vi "Test Set Subpanels-- SMO Array -- Started -- Duplicates.vi"(8 "error in":errorcluster) -> (0 "error out":errorcluster)   [LabVIEW 2020]
uses:
  Maui 2.0/Maui 2.0.lvclass
  C:/Program Files (x86)/National Instruments/LabVIEW 2020/vi.lib/JKI/JKI SMO/SMO/SMO.lvclass
  <vilib>/addons/_JKI Toolkits/Caraya/classes/Assert/Assert Equal Value_Variant.vi
  <vilib>/addons/_JKI Toolkits/Caraya/classes/Test/Test.lvclass
  <vilib>/JKI/JKI SMO/SMO/SMO.lvclass
  C:/Users/Albro/Documents/GitHub/MAUI-Engine/lvsrc/Maui 2.0/Maui 2.0/Maui 2.0.lvclass
  <vilib>/addons/_JKI Toolkits/Caraya/classes/Assert/Assert.lvclass
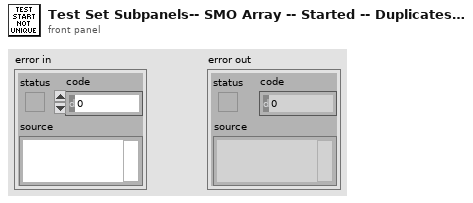
[diagram p1: front panel]
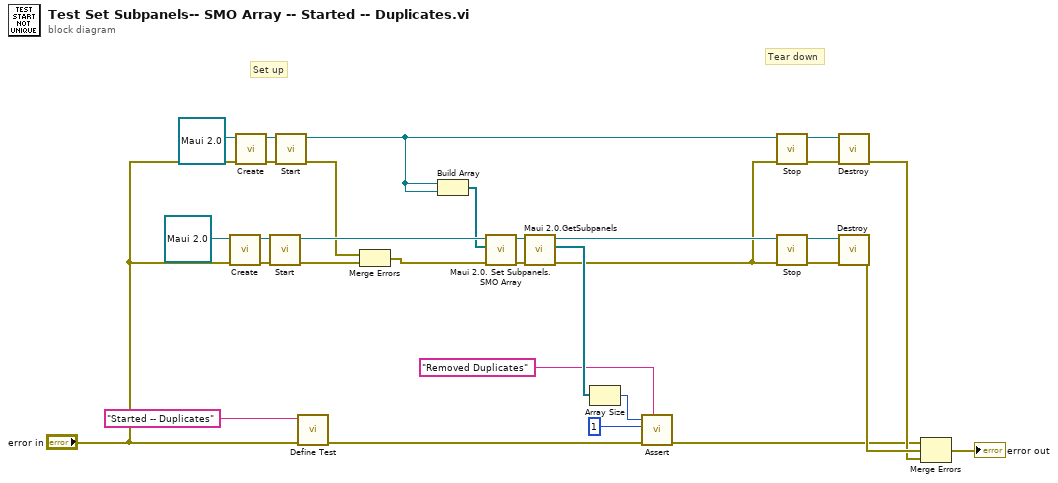
[diagram p0: block diagram]
diagram:
  # "Tear down"
  # "Set up"
  n1 = call <vilib>:"Create.vi"("error in (no error)"="error in", "SMO"=refnum<class "Maui 2.0.lvclass"> refnum ("Maui 2.0.lvclass")) -> ("error out"=w29:errorcluster, "SMO out"=w28:refnum<class "Maui 2.0.lvclass">)  [unwired: 7 in, 1 out]
  n2 = call <vilib>:"Create.vi"("error in (no error)"="error in", "SMO"=refnum<class "Maui 2.0.lvclass"> refnum ("Maui 2.0.lvclass")) -> ("error out"=w19:errorcluster, "SMO out"=w20:refnum<class "Maui 2.0.lvclass">)  [unwired: 7 in, 1 out]
  n3 = call <vilib>:"Start.vi"("error in (no error)"=w29, "SMO"=w28) -> ("error out"=w2:errorcluster, "SMO out"=w26:refnum<class "Maui 2.0.lvclass">)  [unwired: 8 in]
  n4 = call <vilib>:"Start.vi"("error in (no error)"=w19, "SMO"=w20) -> ("error out"=w3:errorcluster, "SMO out"=w12:refnum<class "Maui 2.0.lvclass">)  [unwired: 8 in]
  n5 = call <vilib>:"Define Test.vi"("error in (no error)"="error in", "Label (VI Title)"="Started -- Duplicates") -> ("error out"=w18:errorcluster)  [unwired: 9 in]
  n6 = Merge Errors(w3, w2) -> (w1:errorcluster)
  n7 = Build Array(w12, w12) -> (w13:refnum<class "Maui 2.0.lvclass">[])
  n8 = call-dynamic "Maui 2.0. Set Subpanels.SMO Array.vi"("error in (no error)"=w1, "Subpanels"=w13, "Maui 2.0 in"=w26) -> ("error out"=w15:errorcluster, "Maui 2.0 out"=w17:refnum<class "Maui 2.0.lvclass">)  [unwired: 6 in, 1 out]
  n9 = call "Maui 2.0.GetSubpanels.vi"("error in (no error)"=w15, "Maui 2.0"=w17) -> ("error out"=w4:errorcluster, "Subpanels"=w11:refnum<class "SMO.lvclass">[], "Maui 2.0 out"=w16:refnum<class "Maui 2.0.lvclass">)  [unwired: 7 in]
  n10 = Array Size(array=w11) -> (size(s)=w7:i32)
  n11 = call-poly <vilib>:"Assert.vi"("Label"="Removed Duplicates", "error in (no error)"=w18, "Y"=1 ("size(s)"), "X"=w7) -> ("error out"=w5:errorcluster)  [unwired: 7 in]
  n12 = call <vilib>:"Stop.vi"("error in (no error)"=w4, "SMO"=w12) -> ("error out"=w9:errorcluster, "SMO out"=w10:refnum<class "Maui 2.0.lvclass">)  [unwired: 8 in]
  n13 = call <vilib>:"Stop.vi"("error in (no error)"=w4, "SMO"=w16) -> ("error out"=w25:errorcluster, "SMO out"=w24:refnum<class "Maui 2.0.lvclass">)  [unwired: 8 in]
  n14 = call <vilib>:"Destroy.vi"("error in (no error)"=w9, "SMO"=w10) -> ("error out"=w22:errorcluster)  [unwired: 9 in]
  n15 = call <vilib>:"Destroy.vi"("error in (no error)"=w25, "SMO"=w24) -> ("error out"=w23:errorcluster)  [unwired: 9 in]
  n16 = Merge Errors(w5, w23, w22) -> (→"error out":errorcluster)
